vi "StructureWithLabel.vi"   [LabVIEW 2017]
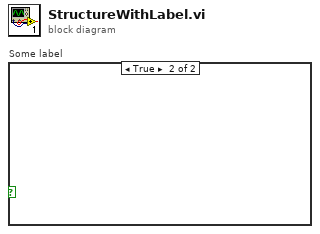
[diagram p0: block diagram]
diagram:
  n1 = case "Some label" shown="True" {
    selector: _ -> [_ _]
    frame False {
    }
    frame True {
    }
  }
